vi "Get Sync Refnums.vi"(8 "error in (no error)":errorcluster, 9 "Module ID":i32) -> (0 "error out":errorcluster, 1 "Stop Sync":T1, 2 "Event Sync":T1, 3 "Module Sync":T1)   [LabVIEW 2018, in "CE14_v2.lvlib"]
doc: "Create or obtain the sync refnums used to synchronize event generation, event registration and stop module between the module clone(s) and its caller(s).\n_____\nBased on DQMH Project Template 6.0.0.91."
uses:
  CE14_v2.lvlib
  Clone Registration/Clone Registration.lvlib
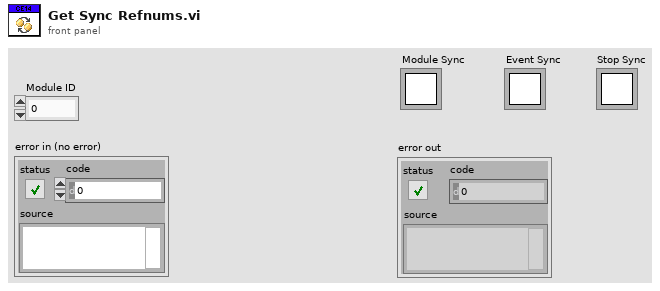
[diagram p1: front panel]
types:
  T1 = typedef "Rendezvous RefNum" = refnum<k1>
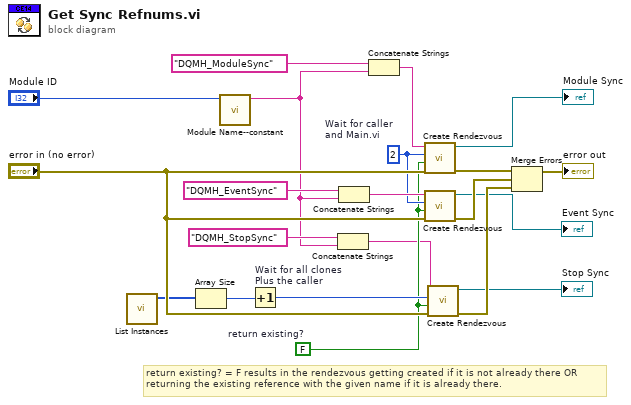
[diagram p0: block diagram]
diagram:
  w5 = FALSE  # return existing?
  w9 = 2  # Wait for caller and Main.vi
  # "return existing? = F results in the rendezvous getting created if it is not already there OR\nreturning the existing reference with the given name if it is already there."
  n1 = call "List Instances.vi"() -> ("Module IDs"=w7:i32[])  [unwired: 7 in, 4 out]
  n2 = Array Size(array=w7) -> (size(s)=w8:i32)
  n3 = call "Module Name--constant.vi"("Module ID"="Module ID") -> ("Module Name"=w2:string)  [unwired: 10 in]
  n4 = Increment "Wait for all clones\nPlus the caller"(x=w8) -> (x+1=w6:i32)
  n5 = Concatenate Strings("DQMH_StopSync" ("name (unnamed)"), w2) -> (w1:string)
  n6 = Concatenate Strings("DQMH_EventSync" ("name (unnamed)"), w2) -> (w11:string)
  n7 = Concatenate Strings("DQMH_ModuleSync" ("name (unnamed)"), w2) -> (w13:string)
  n8 = call <vilib>:"Create Rendezvous.vi"("error in (no error)"="error in (no error)", "return existing (F)"=w5, "size (2)"=w9, "name (unnamed)"=w13) -> ("error out"=w15:errorcluster, "rendezvous"=→"Module Sync":T1)  [unwired: 1 in, 1 out]
  n9 = call <vilib>:"Create Rendezvous.vi"("error in (no error)"="error in (no error)", "return existing (F)"=w5, "size (2)"=w9, "name (unnamed)"=w11) -> ("error out"=w20:errorcluster, "rendezvous"=→"Event Sync":T1)  [unwired: 1 in, 1 out]
  n10 = call <vilib>:"Create Rendezvous.vi"("error in (no error)"="error in (no error)", "return existing (F)"=w5, "size (2)"=w6, "name (unnamed)"=w1) -> ("error out"=w19:errorcluster, "rendezvous"=→"Stop Sync":T1)  [unwired: 1 in, 1 out]
  n11 = Merge Errors(w15, w20, w19) -> (→"error out":errorcluster)
